vi "the_greatest.vi"(2 "T1":dbl, 3 "T2 + D":dbl) -> (7 "max":dbl)   [LabVIEW 2015]
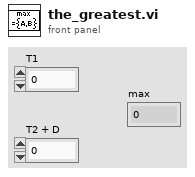
[diagram p1: front panel]
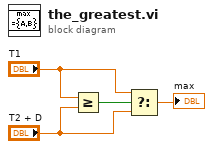
[diagram p0: block diagram]
diagram:
  n1 = Greater Or Equal?(x="T1", y="T2 + D") -> (x >= y?=w1:bool)
  n2 = Select(t="T1", s=w1, f="T2 + D") -> (s? t:f=→"max":dbl)
